vi "Global.vi"() -> ()   [LabVIEW 2014]
panel:
  in  "Boolean":bool
  in  "Config Data":T1
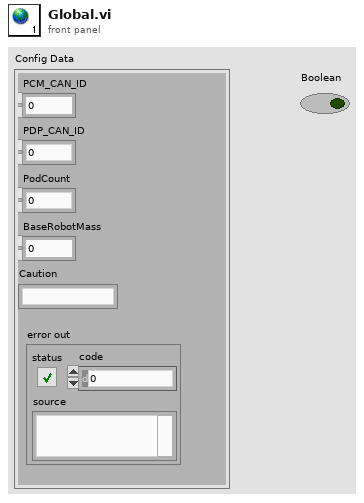
[diagram p1: front panel]
types:
  T1 = cluster{"PCM_CAN_ID":dbl, "PDP_CAN_ID":dbl, "PodCount":dbl, "BaseRobotMass":dbl, "Caution":string, "error out":errorcluster}
diagram:
